vi "enableMotion.vi"(8 "error in (no error)":errorcluster, 10 "model":refnum<class "Model.lvclass">, 11 "StoppedState in":refnum<class "StoppedState.lvclass">) -> (0 "error out":errorcluster, 2 "model 2":refnum<class "Model.lvclass">, 3 "StoppedState out":refnum<class "StoppedState.lvclass">)   [LabVIEW 2013, in "StoppedState.lvclass"]
uses:
  StoppedState.lvclass
  EnabledState/EnabledState.lvclass
  Model/Model/Model.lvclass
  Typedefs/StateSelector.ctl
  Typedefs/M2AADTTypedefs.lvlib
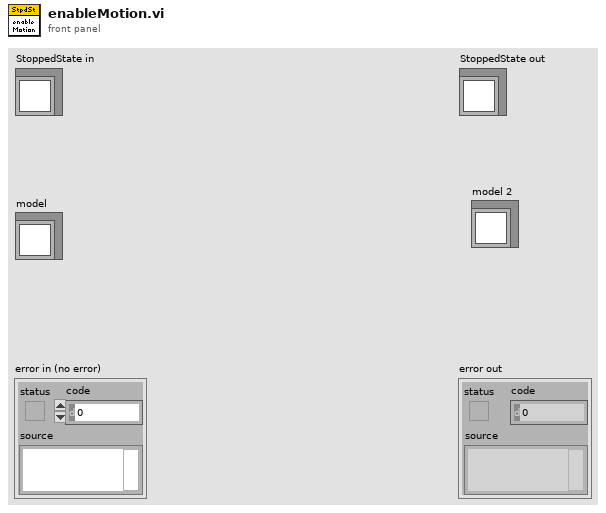
[diagram p1: front panel]
types:
  T1 = typedef "M2AADTTypedefs.lvlib/StateSelector.ctl" = enum16{"EndingCycleState", "FaultState", "InteractiveMotionState", "MovingToNewForceState", "OffState", "PausingState", "StandbyState", "StoppedState"}
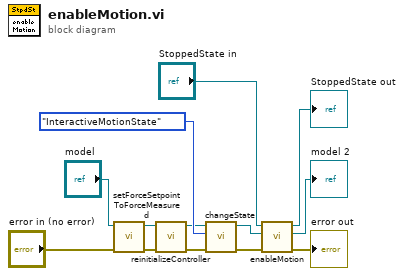
[diagram p0: block diagram]
diagram:
  n1 = call "setForceSetpointToForceMeasured.vi"("error in (no error)"="error in (no error)", "Model in"="model") -> ("error out"=w2:errorcluster, "Model out"=w4:refnum<class "Model.lvclass">)  [unwired: 8 in]
  n2 = call "reinitializeController.vi"("error in (no error)"=w2, "Model in"=w4) -> ("error out"=w1:errorcluster, "Model out"=w3:refnum<class "Model.lvclass">)  [unwired: 8 in]
  n3 = call "changeState.vi"("error in (no error)"=w1, "State:"=StateSelector."InteractiveMotionState", "Model in"=w3) -> ("error out"=w6:errorcluster, "Model out"=w8:refnum<class "Model.lvclass">)  [unwired: 7 in]
  n4 = call-parent "enableMotion.vi"("error in (no error)"=w6, "model"=w8, "State in"="StoppedState in") -> ("error out"=→"error out":errorcluster, "model 2"=→"model 2":refnum<class "Model.lvclass">, "State out"=→"StoppedState out":refnum<class "StoppedState.lvclass">)  [unwired: 6 in]
